vi "Init Scan.vi"(8 "error in (no error)":errorcluster, 10 "Total Steps":u16, 11 "Acq_Scan_Controller_Interface in":refnum<class "Acq_Scan_Controller_Interface.lvclass">) -> (0 "error out":errorcluster, 3 "Acq_Scan_Controller_Interface out":refnum<class "Acq_Scan_Controller_Interface.lvclass">)   [LabVIEW 2023, in "Acq_Scan_Controller_Interface.lvclass"]
uses:
  Acq_Scan_Controller_Interface.lvclass
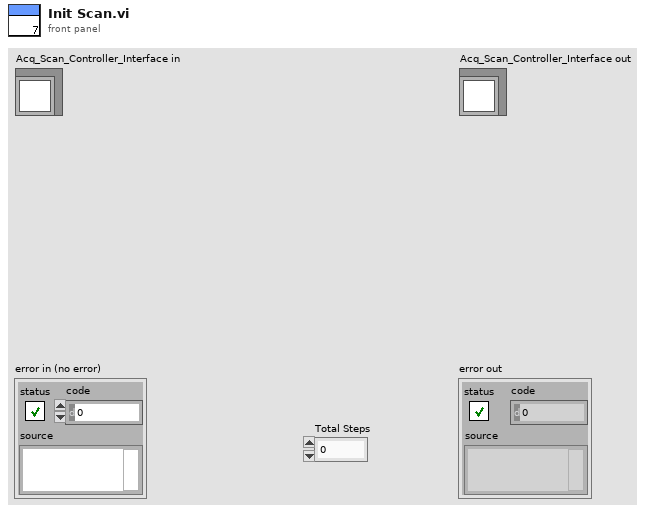
[diagram p1: front panel]
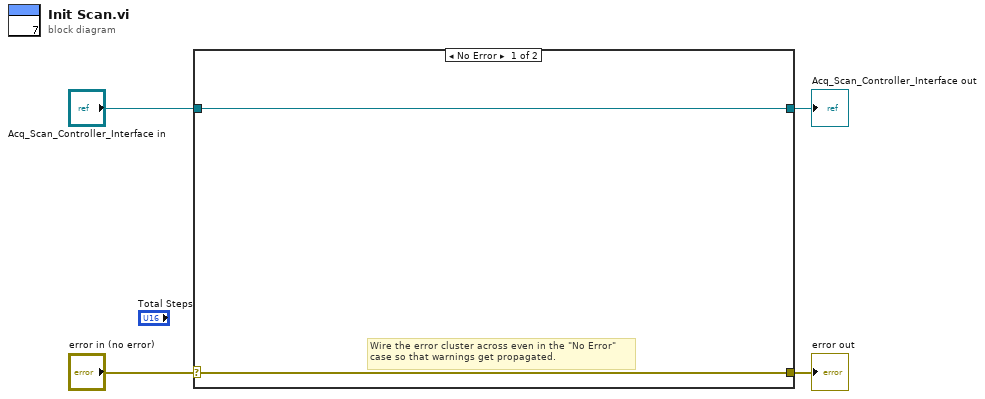
[diagram p0: block diagram]
diagram:
  n1 = case shown="No Error" "error in (no error)" {
    selector: "error in (no error)" -> [w5 w8]
    tunnel: [w5 w8] -> w3
    tunnel: [w6 w7] -> w1
    tunnel: "Acq_Scan_Controller_Interface in" -> [w6 w7]
    frame No Error {
      # "Wire the error cluster across even in the \"No Error\"\ncase so that warnings get propagated."
    }
    frame Error {
    }
  }
  "error out" <- w3
  "Acq_Scan_Controller_Interface out" <- w1
